vi "Launch Mediator Bus Monitor.vi"(8 "error in (no error)":errorcluster, 10 "MediatorBusMonitor":refnum<class "MediatorBusMonitor.lvclass">, 11 "Mediator in":refnum<class "Mediator.lvclass">) -> (0 "error out":errorcluster, 3 "Mediator out":refnum<class "Mediator.lvclass">)   [LabVIEW 2015, in "Mediator.lvlib" / "Mediator.lvclass"]
uses:
  Mediator.lvclass
  MediatorBusMonitor/MediatorBusMonitor.lvclass
  Mediator.lvclass/Mediator.ctl
  <vilib>/ActorFramework/Message Enqueuer/Message Enqueuer.lvclass/Message Enqueuer.ctl
  <vilib>/ActorFramework/Message Enqueuer/Enqueue.vi
  <vilib>/ActorFramework/Message Priority Queue/Priority Enqueue.vi
  <vilib>/ActorFramework/Stop Msg/Stop Msg.lvclass
  <vilib>/ActorFramework/Actor/Actor.lvclass
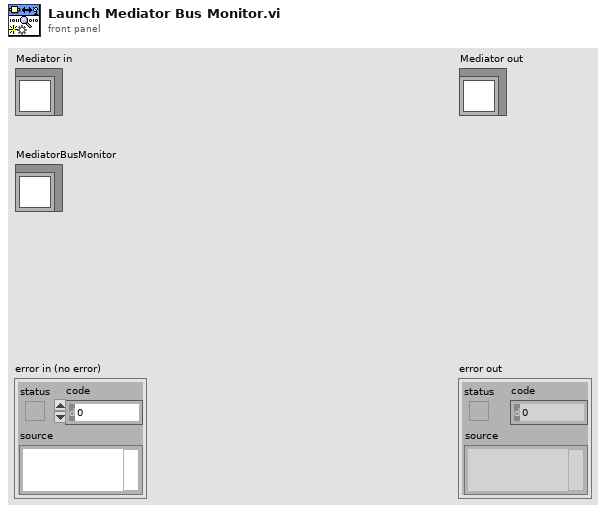
[diagram p1: front panel]
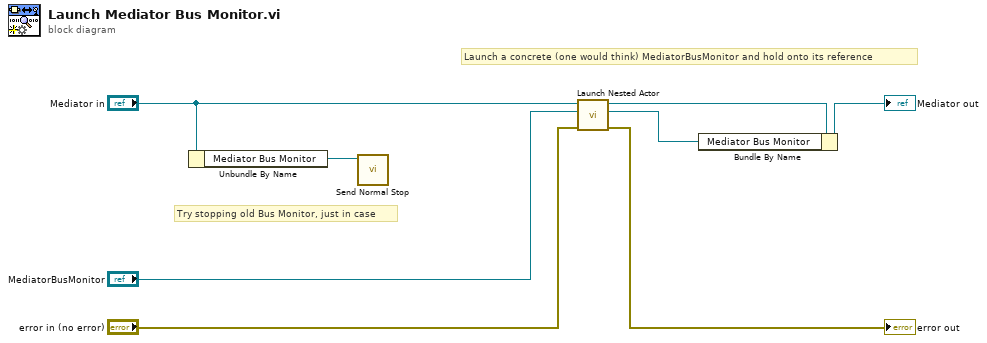
[diagram p0: block diagram]
diagram:
  # "Try stopping old Bus Monitor, just in case"
  # "Launch a concrete (one would think) MediatorBusMonitor and hold onto its reference"
  n1 = Unbundle By Name("Mediator in") -> ("Mediator Bus Monitor"=w1:refnum<class "Message Enqueuer.lvclass">)
  n2 = call <vilib>:"Send Normal Stop.vi"("Message Enqueuer"=w1) -> ()  [unwired: 10 in, 1 out]
  n3 = call <vilib>:"Launch Nested Actor.vi"("error in (no error)"="error in (no error)", "Nested Actor"="MediatorBusMonitor", "Caller Actor in"="Mediator in") -> ("error out"=→"error out":errorcluster, "Nested Actor's Enqueuer"=w3:refnum<class "Message Enqueuer.lvclass">, "Caller Actor out"=w7:refnum<class "Mediator.lvclass">)  [unwired: 6 in]
  n4 = Bundle By Name(cluster=w7, "Mediator Bus Monitor"=w3) -> (→"Mediator out":refnum<class "Mediator.lvclass">)
